vi "Read FIFO.vi"(8 "error in (no error)":errorcluster, 11 "NI_AWS_SQS in":refnum<class "NI_AWS_SQS.lvclass">) -> (0 "error out":errorcluster, 2 "FIFO":bool, 3 "NI_AWS_SQS out":refnum<class "NI_AWS_SQS.lvclass">)   [LabVIEW 2015, in "NI_AWS_SQS.lvclass"]
uses:
  NI_AWS_SQS.lvclass
  NI_AWS_SQS.lvclass/NI_AWS_SQS.ctl
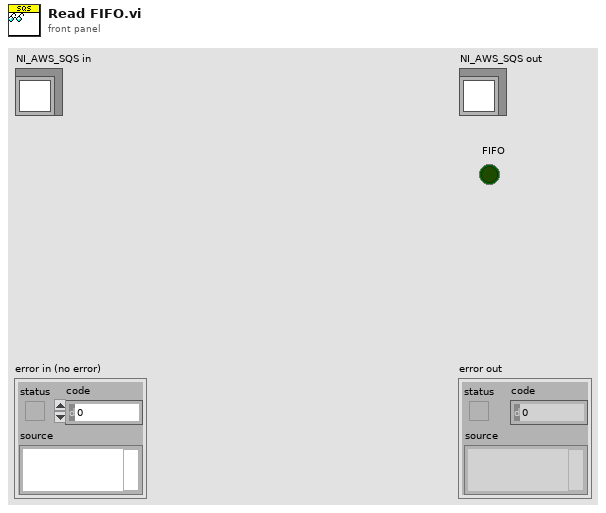
[diagram p1: front panel]
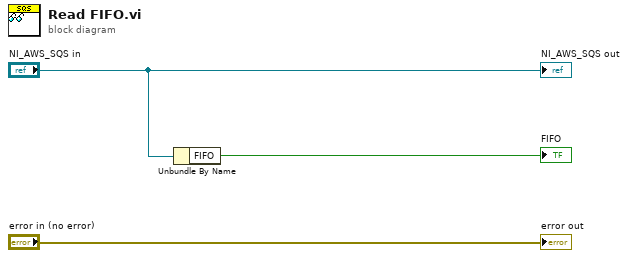
[diagram p0: block diagram]
diagram:
  n1 = Unbundle By Name("NI_AWS_SQS in") -> ("FIFO"=→"FIFO":bool)
  "error out" <- "error in (no error)"
  "NI_AWS_SQS out" <- "NI_AWS_SQS in"
